vi "MultiScanDrift_dev.vi"() -> ()   [LabVIEW 2014]
uses:
  shared/CorrelImages (SubVI)Single.vi
  <userlib>/Nanonis Prog Interface V5/Nanonis Prog Interface.lvlib
panel:
  in  "Multipass":bool=TRUE
  in  "Add":bool
  in  "end":sgl=1.0 format="%#_6p"
  in  "step":sgl=0.05 format="%#_6p"
  in  "start":sgl=-1.5 format="%#_6p"
  in  "create Range":bool
  in  "PLL ON/OFF":bool
  in  "ref bias":dbl=-0.0012 format="%#_6p"
  in  "ref setpoint":bool
  in  "DC On":bool=TRUE
  out "Y drift":i32
  out "X drift":i32
  out "DC active":bool
  in  "Drift correction Pixels":i32=128
  in  "Img Current":sgl=1e-10 format="%#_6p"
  in  "Img Bias (V) DC":sgl=1.0 format="%_2p"
  in  "Forward Speed":sgl=1.2e-09 format="%#_6p"
  in  "Backward Speed":sgl=8e-08 format="%#_6p"
  in  "Img Speed":sgl=4.5e-08 format="%#_6p"
  in  "Channel index (0-23)":u8(ring) items=["Current"=0, "Z (m)"=14]
  in  "Settling time (s)":dbl=0.7 format="%#_6p"
  in  "img bias":bool
  in  "img bias":dbl=-0.0012 format="%#_6p"
  in  "img delay (s)":u32=1
  out "tipLift":dbl format="%#_6p"
  in  "TipLiftList":i32(listbox)
  in  "Const Height":bool
  in  "CurrentList":i32(listbox)
  in  "BiasList":i32(listbox)=35
  out "Current":dbl=5e-11 format="%#_6p"
  out "Bias":dbl=0.02 format="%#_6p"
  # "Turn continuous scan off\n zero tiplift is '0'"
  # "Multipass Windows \nneeds to be open\n and OFF"
  # "5"
  # "10"
  # "15"
  # "20"
  # "25"
  # "30"
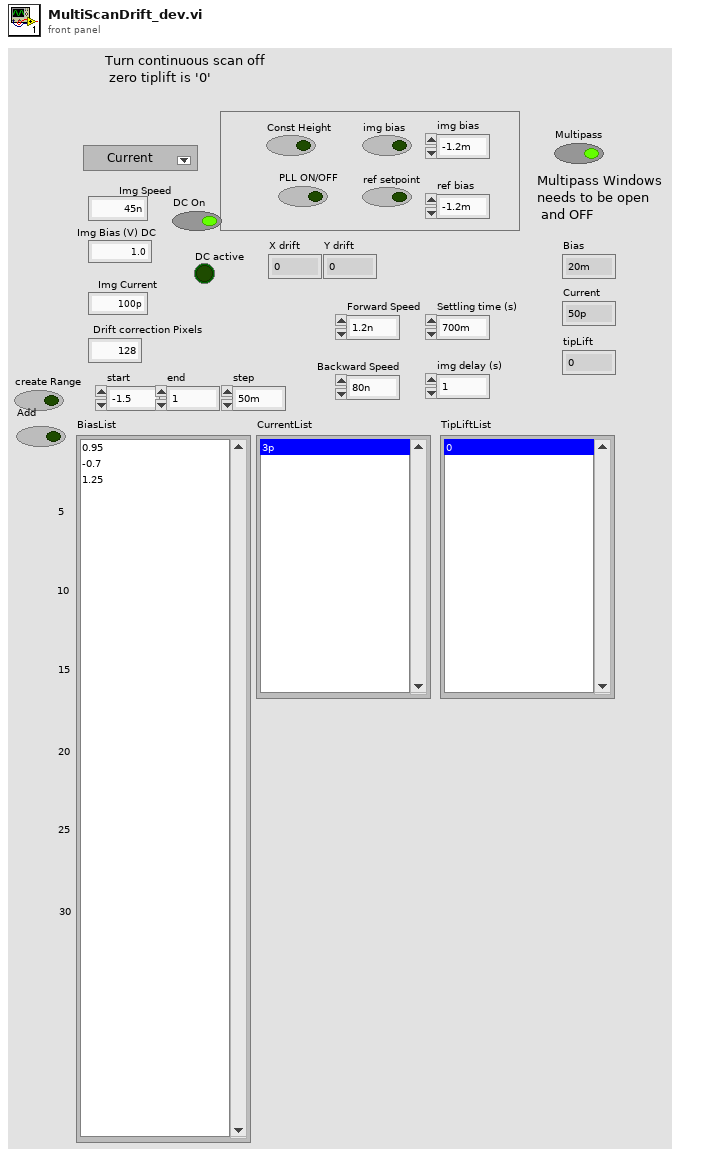
[diagram p1: front panel]
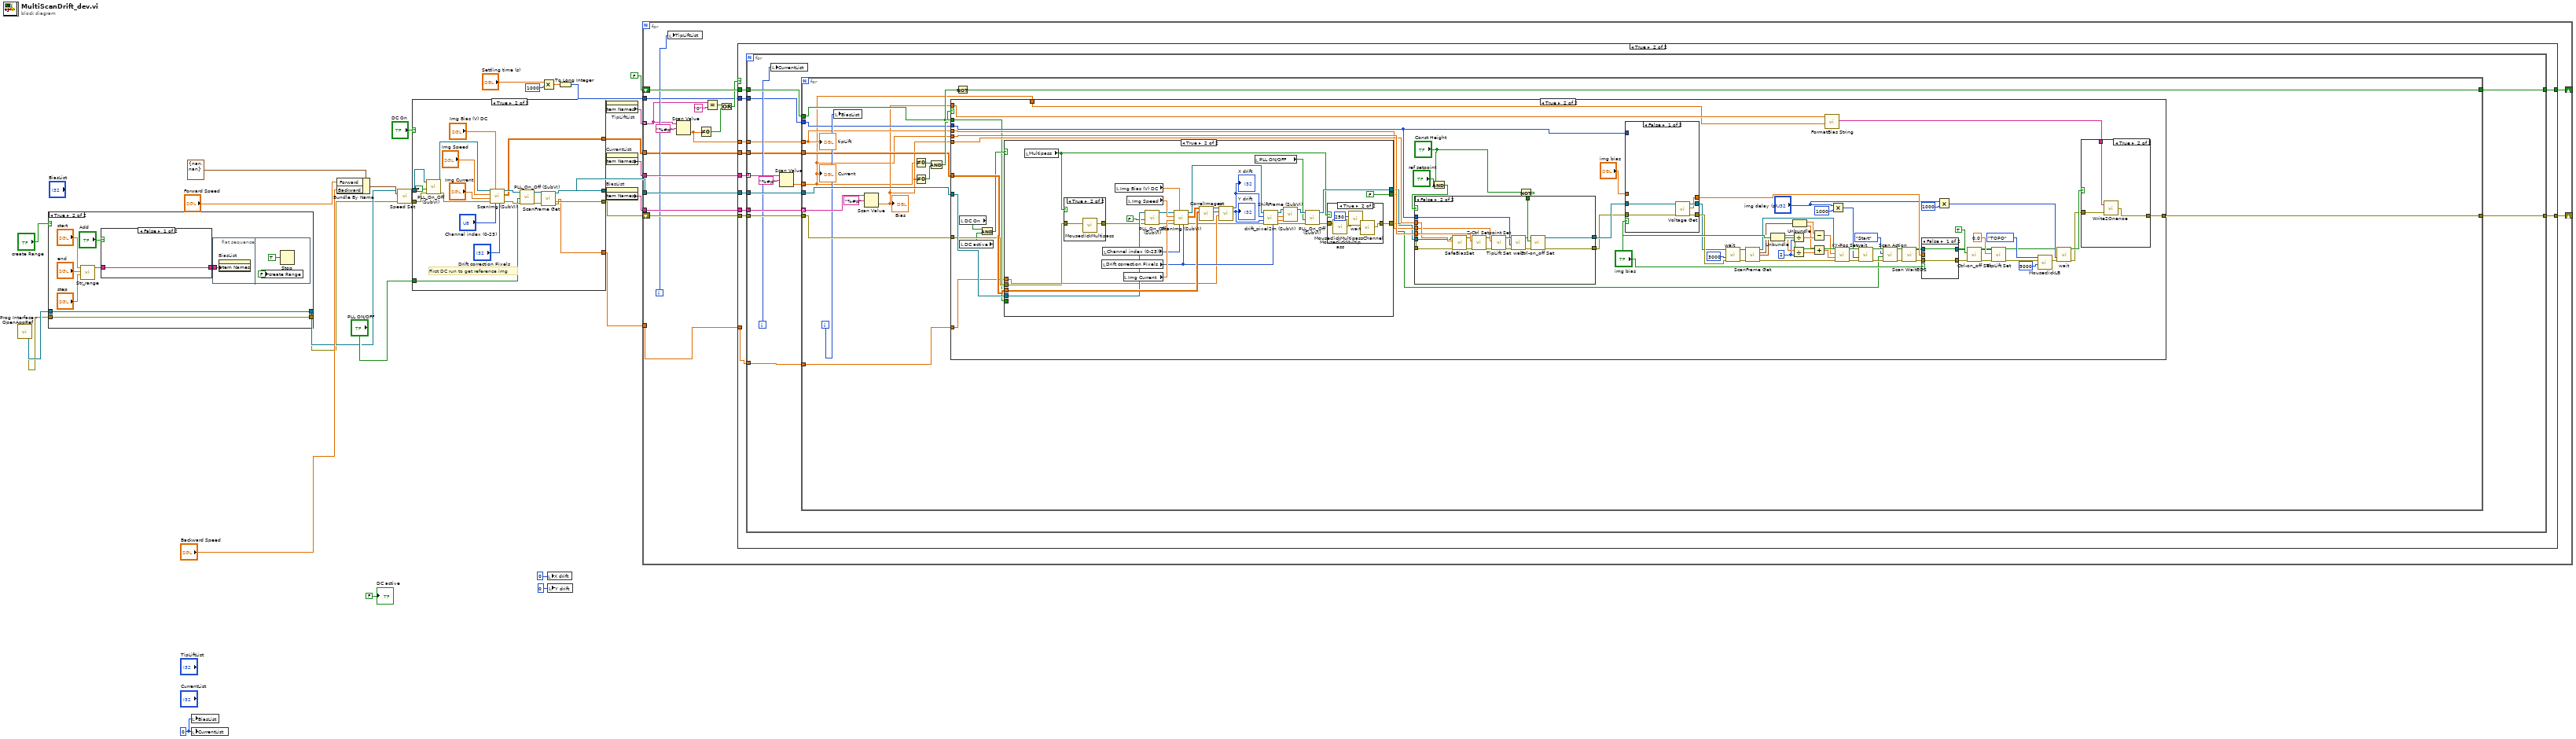
[diagram p0: block diagram]
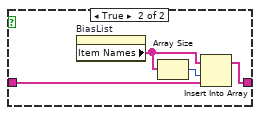
[diagram p3: hidden frame]
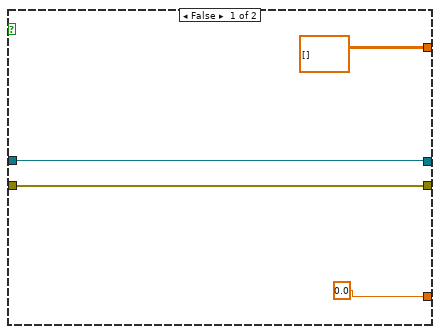
[diagram p4: hidden frame]
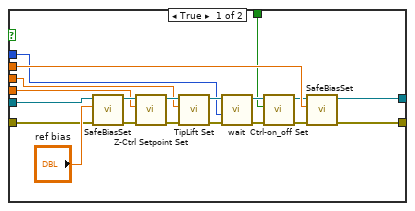
[diagram p7: hidden frame]
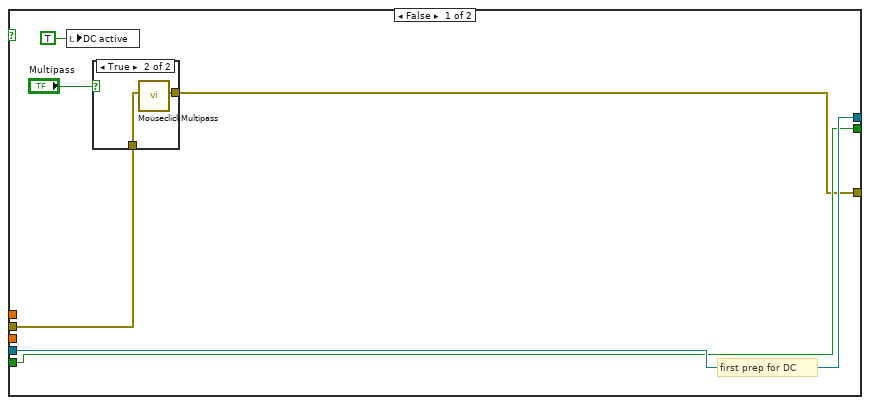
[diagram p9: hidden frame]
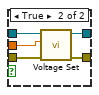
[diagram p13: hidden frame]
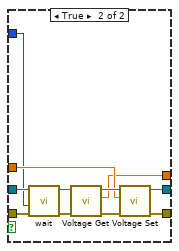
[diagram p14: hidden frame]
diagram:
  w29 = 0 ("BiasList")
  n1 = call <userlib>:"Prog Interface - OpenAppRef.vi"() -> ("Error out"=w2:errorcluster, "Application reference"=w4:refnum<vi>)  [unwired: 6 in]
  n2 = case shown="True" "create Range" {
    tunnel: w4 -> [w31 w39]
    tunnel: [w31 w39] -> w3
    tunnel: w2 -> [w30 w38]
    tunnel: [w30 w38] -> w1
    frame False {
    }
    frame True {
      n3 = call "Str_range.vi"("step"="step", "end"="end", "start"="start") -> ("Item Names"=w32:string[])  [unwired: 8 in]
      n4 = case shown="False" "Add" {
        tunnel: [w43 w45] -> w33
        tunnel: w32 -> [w43 w44]
        frame False {
        }
        frame True {
          n5 = property on="BiasList" class="LstBox (strict)"() -> ("Item Names"=w46:string[])  [unwired: 2 in, 2 out]
          n6 = Array Size(array=w46) -> (size(s)=w47:i32)
          n7 = Insert Into Array(array=w46, index=w47, new element=w44) -> (w45:string[])
        }
      }
      n8 = flat-sequence {
        tunnel: w33 -> [w40]
        frame #0 {
          n9 = property on="BiasList" class="LstBox (strict)"("Item Names"=w40) -> ()  [unwired: 2 in, 2 out]
        }
        frame #1 {
          n10 = local write "create Range"(FALSE ("Range")) -> ()
          n11 = Stop(stop? (T)=TRUE) -> ()
        }
      }
    }
  }
  n12 = local write "BiasList"(w29) -> ()
  n13 = local write "CurrentList"(w29) -> ()
  n14 = Bundle By Name(cluster=cluster{"Forward":sgl, "Backward":sgl} {"Forward"=nan, "Backward"=nan} ("Speed (m/s)"), "Forward"="Forward Speed", "Backward"="Backward Speed") -> (w15:cluster{"Forward":sgl, "Backward":sgl})
  n15 = call <userlib>:"Speed Set.vi"("Application ref in"=w3, "Speed (m/s)"=w15, "error in (no error)"=w1) -> ("Application ref out"=w13:refnum<vi>, "error out"=w12:errorcluster)  [unwired: 11 in]
  n16 = case shown="True" "DC On" {
    tunnel: [w50 w55] -> w17
    tunnel: [w49 w54] -> w16
    tunnel: [dbl[][] [] ("Img") w64] -> w14
    tunnel: w13 -> [w50 w63]
    tunnel: w12 -> [w49 w61]
    tunnel: [sgl 0.0 ("Angle (deg)") w53] -> w7
    tunnel: "PLL ON/OFF" -> [_ w52]
    frame False {
    }
    frame True {
      # "First DC run to get reference img"
      n17 = call "PLL_On_Off (SubVI).vi"("error in (no error)"=w61, "Output ON/OFF (F=OFF)"=FALSE, "Application in"=w63) -> ("error out"=w60:errorcluster, "Application out"=w62:refnum<vi>)  [unwired: 7 in]
      n18 = call "ScanImg (SubVI).vi"("pixel"="Drift correction Pixels", "Channel index (0-23)"="Channel index (0-23)", "Bias (V)"="Img Bias (V) DC", "error in (no error)"=w60, "Current"="Img Current", "Img Speed"="Img Speed", "Application in"=w62) -> ("error out"=w67:errorcluster, "Img"=w64:dbl[][], "Application out"=w68:refnum<vi>)  [unwired: 2 in]
      n19 = call "PLL_On_Off (SubVI).vi"("error in (no error)"=w67, "Output ON/OFF (F=OFF)"=w52, "Application in"=w68) -> ("error out"=w56:errorcluster, "Application out"=w57:refnum<vi>)  [unwired: 7 in]
      n20 = call <userlib>:"ScanFrame Get.vi"("Application ref in"=w57, "error in (no error)"=w56) -> ("Application ref out"=w55:refnum<vi>, "Angle (deg)"=w53:sgl, "error out"=w54:errorcluster)  [unwired: 9 in, 2 out]
    }
  }
  n21 = Multiply(x="Settling time (s)", y=u32 1000) -> (x*y=w25:dbl)
  n22 = local write "X drift"(0 ("X drift")) -> ()
  n23 = local write "Y drift"(0 ("Y drift")) -> ()
  n24 = To Long Integer(number=w25) -> (32bit integer=w26:i32)
  n25 = property on="TipLiftList" class="LstBox (strict)"() -> ("Item Names"=w21:string[])  [unwired: 2 in, 2 out]
  n26 = property on="CurrentList" class="LstBox (strict)"() -> ("Item Names"=w22:string[])  [unwired: 2 in, 2 out]
  n27 = property on="BiasList" class="LstBox (strict)"() -> ("Item Names"=w23:string[])  [unwired: 2 in, 2 out]
  n28 = for {
    tunnel: w23 -> [w87]
    tunnel: w22 -> [w86]
    tunnel: w17 -> [w85]
    tunnel: w21 -> [w81] mode=indexing
    shift-right: [w75] -> _
    shift-left: FALSE ("Direction: up/down (T=up)") -> [w88]
    tunnel: w26 -> [w74]
    tunnel: w14 -> [w73]
    tunnel: w7 -> [w72]
    shift-right: [w71] -> _
    shift-left: w16 -> [w84]
    i -> [w82]
    n29 = local write "TipLiftList"(w82) -> ()
    n30 = Scan Value(string=w81, format string="%#p") -> (value=w80:dbl)  [unwired: 1 in, 1 out]
    n31 = Not Equal To 0?(x=w80) -> (x != 0?=w79:bool)
    n32 = Equal?(x=w81, y="0") -> (x = y?=w76:bool)
    n33 = Or(x=w76, y=w79) -> (x .or. y?=w78:bool)
    n34 = case shown="True" w78 {
      tunnel: w88 -> [w90 w101]
      tunnel: w87 -> [_ w100]
      tunnel: w86 -> [_ w99]
      tunnel: w85 -> [_ w98]
      tunnel: w84 -> [w89 w97]
      tunnel: w80 -> [_ w96]
      tunnel: [w90 w95] -> w75
      tunnel: w74 -> [_ w94]
      tunnel: w73 -> [_ w93]
      tunnel: w72 -> [_ w92]
      tunnel: [w89 w91] -> w71
      frame False {
      }
      frame True {
        n35 = for {
          tunnel: w101 -> [w115]
          tunnel: w98 -> [w114]
          tunnel: w97 -> [w113]
          tunnel: w100 -> [w112]
          tunnel: w99 -> [w110] mode=indexing
          tunnel: w96 -> [w107]
          tunnel: [w106] -> w95
          tunnel: w94 -> [w105]
          tunnel: w93 -> [w104]
          tunnel: w92 -> [w103]
          tunnel: [w102] -> w91
          i -> [w108]
          n36 = local write "CurrentList"(w108) -> ()
          n37 = Scan Value(string=w110, format string="%#p") -> (value=w109:dbl)  [unwired: 1 in, 1 out]
          n38 = for {
            tunnel: w112 -> [w127] mode=indexing
            tunnel: w114 -> [w129]
            tunnel: w113 -> [w128]
            tunnel: w109 -> [w117]
            tunnel: w107 -> [w122]
            tunnel: w115 -> [w131]
            tunnel: [w130] -> w106
            tunnel: w105 -> [w121]
            tunnel: w104 -> [w120]
            tunnel: w103 -> [w119]
            tunnel: [w116] -> w102
            i -> [w123]
            n39 = local write "BiasList"(w123) -> ()
            n40 = Scan Value(string=w127, format string="%#p") -> (value=w118:dbl)  [unwired: 1 in, 1 out]
            "Bias" <- w118
            n41 = Not Equal To 0?(x=w117) -> (x != 0?=w126:bool)
            n42 = Not Equal To 0?(x=w118) -> (x != 0?=w125:bool)
            n43 = Compound Arithmetic op=AND(w126, w125) -> (w124:bool)
            n44 = case shown="True" w124 {
              tunnel: w131 -> [_ w173]
              tunnel: w118 -> [_ w203]
              tunnel: w129 -> [_ w180]
              tunnel: w128 -> [w133 w179]
              tunnel: w117 -> [_ w204]
              tunnel: w122 -> [_ w200]
              tunnel: w121 -> [_ w182]
              tunnel: w120 -> [_ w181]
              tunnel: w119 -> [_ w172]
              tunnel: w118 -> [_ w171]
              tunnel: w117 -> [_ w170]
              tunnel: [w133 w166] -> w116
              frame False {
              }
              frame True {
                w151 = 2
                n45 = local read "DC On"() -> (w175:bool)
                n46 = local read "DC active"() -> (w176:bool)
                n47 = And(x=w175, y=w176) -> (x .and. y?=w174:bool)
                n48 = case shown="True" w174 {
                  tunnel: w181 -> [_ w285]
                  tunnel: w180 -> [w251 w275]
                  tunnel: w179 -> [w247 w262]
                  tunnel: [w246 w256] -> w178
                  tunnel: [w251 w272] -> w177
                  tunnel: [w249 FALSE ("Direction: up/down (T=up)")] -> w136
                  tunnel: w173 -> [w249 _]
                  tunnel: w172 -> [_ w268]
                  frame False {
                    # "first prep for DC"
                    n49 = local write "DC active"(TRUE ("DC active")) -> ()
                    n50 = case shown="True" "Multipass" {
                      tunnel: w247 -> [w252 w254]
                      tunnel: [w252 w253] -> w246
                      frame False {
                      }
                      frame True {
                        n51 = call "MouseclickMultipass.vi"("error in (no error)"=w254) -> ("error out"=w253:errorcluster)  [unwired: 10 in]
                      }
                    }
                  }
                  frame True {
                    n52 = local read "Multipass"() -> (w255:bool)
                    n53 = case shown="True" w255 {
                      tunnel: w262 -> [w292 w294]
                      tunnel: [w292 w293] -> w261
                      frame False {
                      }
                      frame True {
                        n54 = call "MouseclickMultipass.vi"("error in (no error)"=w294) -> ("error out"=w293:errorcluster)  [unwired: 10 in]
                      }
                    }
                    n55 = local read "Drift correction Pixels"() -> (w270:i32)
                    n56 = local read "Channel index (0-23)"() -> (w280:u8)
                    n57 = local read "Img Bias (V) DC"() -> (w281:sgl)
                    n58 = local read "Img Current"() -> (w282:sgl)
                    n59 = local read "Img Speed"() -> (w283:sgl)
                    n60 = call "PLL_On_Off (SubVI).vi"("error in (no error)"=w261, "Output ON/OFF (F=OFF)"=FALSE, "Application in"=w275) -> ("error out"=w260:errorcluster, "Application out"=w274:refnum<vi>)  [unwired: 7 in]
                    n61 = call "ScanImg (SubVI).vi"("pixel"=w270, "Channel index (0-23)"=w280, "Bias (V)"=w281, "error in (no error)"=w260, "Current"=w282, "Img Speed"=w283, "Application in"=w274) -> ("error out"=w259:errorcluster, "Img"=w284:dbl[][], "Application out"=w276:refnum<vi>)  [unwired: 2 in]
                    n62 = call-poly "CorrelImages.vi"("Ref Array"=w285, "New Image"=w284) -> ("Y drift"=w265:i32, "X drift"=w267:i32)  [unwired: 6 in, 2 out]
                    n63 = call "rot.vi"("angle"=w268, "y"=w265, "x"=w267) -> ("y'"=w264:i32, "x'"=w266:i32)  [unwired: 7 in]
                    "X drift" <- w266
                    "Y drift" <- w264
                    n64 = local read "PLL ON/OFF"() -> (w263:bool)
                    n65 = call "drift_pixel2m (SubVI).vi"("Application in"=w276, "X drift"=w266, "Y drift"=w264, "error in"=w259, "Drift correction Pixels"=w270) -> ("Application out"=w277:refnum<vi>, "x drift"=w279:sgl, "y drift"=w278:sgl, "error out"=w258:errorcluster)  [unwired: 1 in]
                    n66 = call "ShiftFrame (SubVI).vi"("Y shift"=w278, "X shift"=w279, "Application in"=w277) -> ("Application out"=w273:refnum<vi>)  [unwired: 8 in]
                    n67 = call "PLL_On_Off (SubVI).vi"("error in (no error)"=w258, "Output ON/OFF (F=OFF)"=w263, "Application in"=w273) -> ("error out"=w257:errorcluster, "Application out"=w272:refnum<vi>)  [unwired: 7 in]
                    n68 = case shown="True" w255 {
                      tunnel: w257 -> [w286 w291]
                      tunnel: [w286 w290] -> w256
                      frame False {
                      }
                      frame True {
                        n69 = call "MouseclickMultipass.vi"("error in (no error)"=w291) -> ("error out"=w289:errorcluster)  [unwired: 10 in]
                        n70 = call "wait.vi"("error in"=w289, "milliseconds to wait"=u32 250) -> ("error out"=w288:errorcluster)  [unwired: 8 in, 1 out]
                        n71 = call "MouseclickMultipassChannel.vi"("error in (no error)"=w288) -> ("error out"=w290:errorcluster)  [unwired: 10 in]
                      }
                    }
                  }
                }
                n72 = And(x="Const Height", y="ref setpoint") -> (x .and. y?=w163:bool)
                n73 = Not(x="Const Height") -> (.not. x?=w202:bool)
                n74 = case shown="False" w163 {
                  tunnel: w204 -> [w211 w241]
                  tunnel: w203 -> [w224 w240]
                  tunnel: w202 -> [w218 w239]
                  tunnel: w200 -> [w212 w237]
                  tunnel: [w206 w236] -> w197
                  tunnel: [w205 w235] -> w196
                  tunnel: w182 -> [w213 w231]
                  tunnel: w178 -> [w209 w230]
                  tunnel: w177 -> [w210 w229]
                  frame True {
                    n75 = call "SafeBiasSet.vi"("Application ref in"=w210, "Bias (V)"="ref bias", "error in (no error)"=w209) -> ("Application ref out"=w221:refnum<vi>, "Error out"=w223:errorcluster)  [unwired: 6 in]
                    n76 = call <userlib>:"Z-Ctrl Setpoint Set.vi"("error in (no error)"=w223, "Z Controller setpoint"=w211, "Application ref in"=w221) -> ("error out"=w215:errorcluster, "Application ref out"=w217:refnum<vi>)  [unwired: 7 in]
                    n77 = call <userlib>:"TipLift Set.vi"("error in (no error)"=w215, "TipLift (m)"=w212, "Application ref in"=w217) -> ("error out"=w214:errorcluster, "Application ref out"=w216:refnum<vi>)  [unwired: 7 in]
                    n78 = call "wait.vi"("error in"=w214, "milliseconds to wait"=w213, "application reference in"=w216) -> ("error out"=w220:errorcluster, "application reference out"=w219:refnum<vi>)  [unwired: 7 in]
                    n79 = call <userlib>:"Ctrl-on_off Set.vi"("error in (no error)"=w220, "Z Controller ON/OFF"=w218, "Application ref in"=w219) -> ("error out"=w207:errorcluster, "Application ref out"=w208:refnum<vi>)  [unwired: 7 in]
                    n80 = call "SafeBiasSet.vi"("Application ref in"=w208, "Bias (V)"=w224, "error in (no error)"=w207) -> ("Application ref out"=w206:refnum<vi>, "Error out"=w205:errorcluster)  [unwired: 6 in]
                  }
                  frame False {
                    n81 = call "SafeBiasSet.vi"("Application ref in"=w229, "Bias (V)"=w240, "error in (no error)"=w230) -> ("Application ref out"=w228:refnum<vi>, "Error out"=w227:errorcluster)  [unwired: 6 in]
                    n82 = call <userlib>:"Z-Ctrl Setpoint Set.vi"("error in (no error)"=w227, "Z Controller setpoint"=w241, "Application ref in"=w228) -> ("error out"=w225:errorcluster, "Application ref out"=w226:refnum<vi>)  [unwired: 7 in]
                    n83 = call <userlib>:"TipLift Set.vi"("error in (no error)"=w225, "TipLift (m)"=w237, "Application ref in"=w226) -> ("error out"=w232:errorcluster, "Application ref out"=w238:refnum<vi>)  [unwired: 7 in]
                    n84 = call "wait.vi"("error in"=w232, "milliseconds to wait"=w231, "application reference in"=w238) -> ("error out"=w233:errorcluster, "application reference out"=w234:refnum<vi>)  [unwired: 7 in]
                    n85 = call <userlib>:"Ctrl-on_off Set.vi"("error in (no error)"=w233, "Z Controller ON/OFF"=w239, "Application ref in"=w234) -> ("error out"=w235:errorcluster, "Application ref out"=w236:refnum<vi>)  [unwired: 7 in]
                  }
                }
                n86 = case shown="False" "img bias" {
                  tunnel: w197 -> [w306 w308]
                  tunnel: [w305 w315] -> w134
                  tunnel: w196 -> [w302 w311]
                  tunnel: [w303 w314] -> w135
                  tunnel: "img bias" -> [_ w313]
                  tunnel: [w304 w312] -> w194
                  tunnel: w182 -> [_ w307]
                  frame False {
                    n87 = call <userlib>:"Voltage Get.vi"("error in (no error)"=w302, "Application ref in"=w306) -> ("error out"=w303:errorcluster, "Bias (V)"=w304:sgl, "Application ref out"=w305:refnum<vi>)  [unwired: 7 in]
                  }
                  frame True {
                    n88 = call "wait.vi"("error in"=w311, "milliseconds to wait"=w307, "application reference in"=w308) -> ("error out"=w310:errorcluster, "application reference out"=w309:refnum<vi>)  [unwired: 7 in]
                    n89 = call <userlib>:"Voltage Get.vi"("error in (no error)"=w310, "Application ref in"=w309) -> ("error out"=w317:errorcluster, "Bias (V)"=w312:sgl, "Application ref out"=w316:refnum<vi>)  [unwired: 7 in]
                    n90 = call <userlib>:"Voltage Set.vi"("Error in (no error)"=w317, "Bias (V)"=w313, "Application ref in"=w316) -> ("Error out"=w314:errorcluster, "Application ref out"=w315:refnum<vi>)  [unwired: 7 in]
                  }
                }
                n91 = call "wait.vi"("error in"=w135, "milliseconds to wait"=u32 3000 ("y"), "application reference in"=w134) -> ("error out"=w143:errorcluster, "application reference out"=w142:refnum<vi>)  [unwired: 7 in]
                n92 = call <userlib>:"ScanFrame Get.vi"("Application ref in"=w142, "error in (no error)"=w143) -> ("Application ref out"=w162:refnum<vi>, "Center coordinates (m)"=w146:cluster{"Xc":sgl, "Yc":sgl}, "Size (m)"=w147:cluster{"Width":sgl, "Height":sgl}, "error out"=w161:errorcluster)  [unwired: 9 in, 1 out]
                n93 = Unbundle(w147) -> ("Width"=w149:sgl, "Height"=w150:sgl)
                n94 = Divide(x=w149, y=w151) -> (x/y=w153:sgl)
                n95 = Divide(x=w150, y=w151) -> (x/y=w152:sgl)
                n96 = Unbundle(w146) -> ("Xc"=w154:sgl, "Yc"=w148:sgl)
                n97 = Subtract(x=w154, y=w153) -> (x-y=w155:sgl)
                n98 = Add(x=w148, y=w152) -> (x+y=w156:sgl)
                n99 = call "FormatBias String.vi"("current"=w170, "bias"=w171) -> ("resulting string"=w167:string)  [unwired: 9 in]
                n100 = Multiply(x="img delay (s)", y=u32 1000) -> (x*y=w158:u32)
                n101 = call <userlib>:"XY-Pos Set.vi"("error in (no error)"=w161, "Y (m)"=w156, "X (m)"=w155, "Application ref in"=w162) -> ("error out"=w160:errorcluster, "Application ref out"=w159:refnum<vi>)  [unwired: 4 in]
                n102 = call "wait.vi"("error in"=w160, "milliseconds to wait"=w158, "application reference in"=w159) -> ("error out"=w140:errorcluster, "application reference out"=w141:refnum<vi>)  [unwired: 7 in]
                n103 = call <userlib>:"Scan Action.vi"("error in (no error)"=w140, "Direction: up/down (T=up)"=w136, "Scan action (Start)"=enum16{"Start", "Stop", "Pause", "Resume"}."Start", "Application ref in"=w141) -> ("error out"=w138:errorcluster, "Application ref out"=w139:refnum<vi>)  [unwired: 5 in]
                n104 = call <userlib>:"Scan WaitEOS.vi"("error in (no error)"=w138, "Application ref in"=w139) -> ("error out"=w192:errorcluster, "Application ref out"=w193:refnum<vi>)  [unwired: 5 in, 2 out]
                n105 = case shown="False" "img bias" {
                  tunnel: w193 -> [w296 w299]
                  tunnel: [w296 w301] -> w191
                  tunnel: [w295 w300] -> w190
                  tunnel: w192 -> [w295 w298]
                  tunnel: w194 -> [_ w297]
                  frame False {
                  }
                  frame True {
                    n106 = call <userlib>:"Voltage Set.vi"("Error in (no error)"=w298, "Bias (V)"=w297, "Application ref in"=w299) -> ("Error out"=w300:errorcluster, "Application ref out"=w301:refnum<vi>)  [unwired: 7 in]
                  }
                }
                n107 = Multiply(x="img delay (s)", y=u32 1000) -> (x*y=w184:u32)
                n108 = call <userlib>:"Ctrl-on_off Set.vi"("error in (no error)"=w190, "Z Controller ON/OFF"=TRUE, "Application ref in"=w191) -> ("error out"=w189:errorcluster, "Application ref out"=w188:refnum<vi>)  [unwired: 7 in]
                n109 = call <userlib>:"TipLift Set.vi"("error in (no error)"=w189, "TipLift (m)"=sgl 0.0, "Application ref in"=w188) -> ("error out"=w199:errorcluster)  [unwired: 7 in, 1 out]
                n110 = call "MouseclickLB.vi"("nMilliseconds"=5000, "error in (no error)"=w199, "Click"=enum16{"Header", "TOPO", "STS", "GRID"}."TOPO") -> ("error out"=w183:errorcluster)  [unwired: 8 in]
                n111 = call "wait.vi"("error in"=w183, "milliseconds to wait"=w184) -> ("error out"=w168:errorcluster)  [unwired: 8 in, 1 out]
                n112 = case shown="True" "img bias" {
                  tunnel: w168 -> [w242 w245]
                  tunnel: w167 -> [_ w244]
                  tunnel: [w242 w243] -> w166
                  frame False {
                  }
                  frame True {
                    n113 = call "Write2Onenoe.vi"("error in (no error)"=w245, "strSendText"=w244) -> ("error out"=w243:errorcluster)
                  }
                }
              }
            }
            n114 = Not(x=w131) -> (.not. x?=w130:bool)
            "Current" <- w117
            "tipLift" <- w122
          }
        }
      }
    }
  }
  "DC active" <- FALSE ("DC active")
